vi "Replace Channel.vi"(6 "Index":i32, 7 "Display State In":T1={"Current Channels Info"=[], "Help Prefix"="", "Max Display Size"=8, "Max Size"=0, "Show Buttons"=TRUE, "Data Valid"=refnum, "Show Range"=FALSE, "Range Items"=[], "Range Index"=[]}, 8 "error in (no error)":errorcluster, 9 "New Channels View":T7[](array[typedef]), 10 "Old Channels View":T7[](array[typedef]), 11 "Channels In":T4) -> (0 "error out":errorcluster, 3 "Channels Out":T4, 5 "Display State Out":T1={"Current Channels Info"=[], "Help Prefix"="", "Max Display Size"=8, "Max Size"=0, "Show Buttons"=TRUE, "Data Valid"=refnum, "Show Range"=FALSE, "Range Items"=[], "Range Index"=[]})   [LabVIEW 2021, in "myRIO Channel List.xctl"]
uses:
  <vilib>/myRIO/Common/Express VI Framework/xctls/myRIO Channel List/myRIO Channel List.xctl
  <vilib>/myRIO/Common/Express VI Framework/xctls/myRIO Channel List/typedefs/Channel View.ctl
  <vilib>/myRIO/Common/Express VI Framework/xctls/myRIO Channel List/typedefs/Error Icon.ctl
  <vilib>/myRIO/Common/Express VI Framework/xctls/myRIO Channel List/typedefs/Remove Channel.ctl
  <vilib>/myRIO/Common/Express VI Framework/xctls/myRIO Channel List/State.ctl
  <vilib>/myRIO/Common/Profile Manager Framework/typedefs/Channel Info.ctl
  <vilib>/myRIO/Common/Express VI Framework/typedefs/Data Validate Ref.ctl
  <vilib>/myRIO/Common/Express VI Framework/xctls/myRIO Channel List/Data.ctl
  <vilib>/myRIO/Common/Express VI Framework/xctls/myRIO Channel List/typedefs/Channel Data.ctl
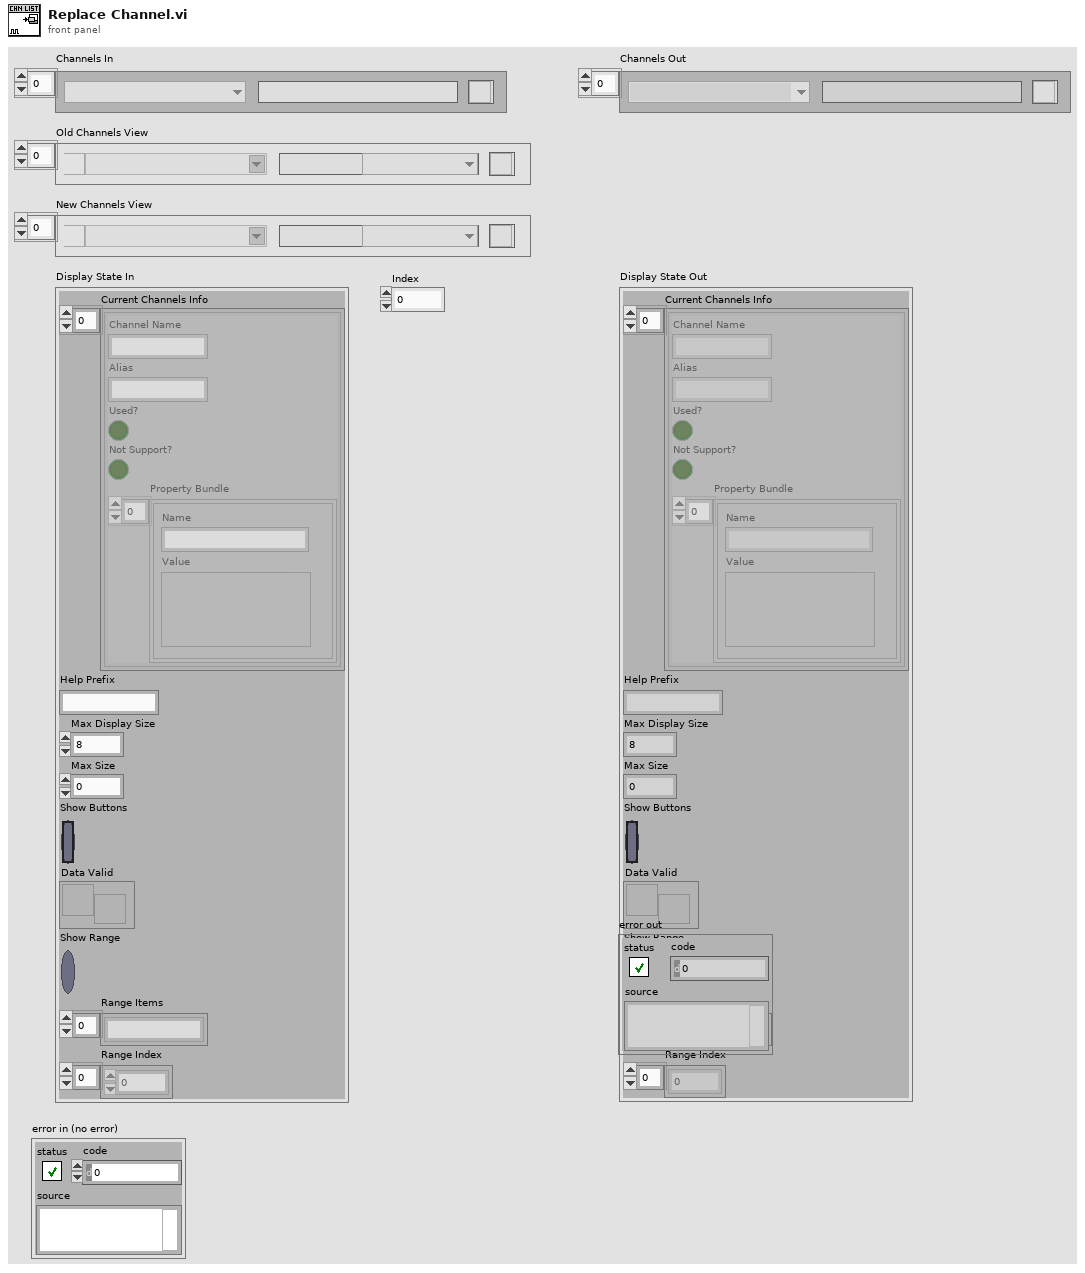
[diagram p1: front panel]
types:
  T1 = typedef "myRIO Channel List.xctl/State.ctl" = cluster{"Current Channels Info":T2[], "Help Prefix":string, "Max Display Size":i32, "Max Size":i32, "Show Buttons":bool, "Data Valid":T3, "Show Range":bool, "Range Items":string[], "Range Index":i32[]}
  T2 = typedef "Channel Info.ctl" = cluster{"Channel Name":string, "Alias":string, "Used?":bool, "Not Support?":bool, "Property Bundle":cluster{"Name":string, "Value":variant}[]}
  T3 = typedef "Data Validate Ref.ctl" = refnum<user-event>
  T4 = typedef "myRIO Channel List.xctl/Data.ctl" = T5[]
  T5 = typedef "myRIO Channel List.xctl/Channel Data.ctl" = cluster{"Channel Name":u16, "Channel Alias":string, "Remove Channel":T6, "Index":i32}
  T6 = typedef "myRIO Channel List.xctl/Remove Channel.ctl" = bool
  T7 = typedef "myRIO Channel List.xctl/Channel View.ctl" = cluster{"Error Icon":T8, "Channel Name":string, "Channel Alias":string, "Remove Channel":T6, "Index":i32, "Range":i32}
  T8 = typedef "myRIO Channel List.xctl/Error Icon.ctl" = bool
  T9 = cluster{"Error Icon":T8, "Channel Name":bool, "Channel Alias":bool, "Remove Channel":T6, "Index":bool, "Range":bool}
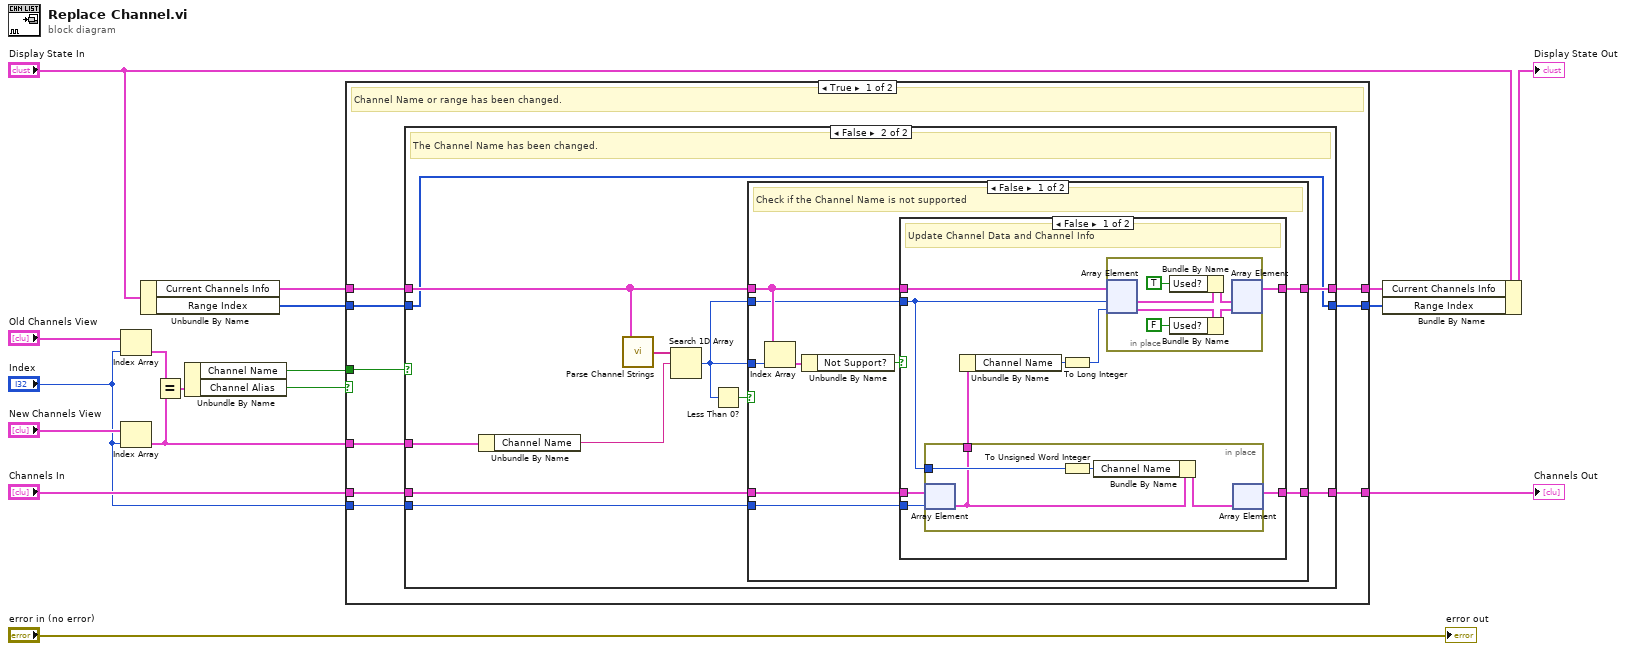
[diagram p0: block diagram]
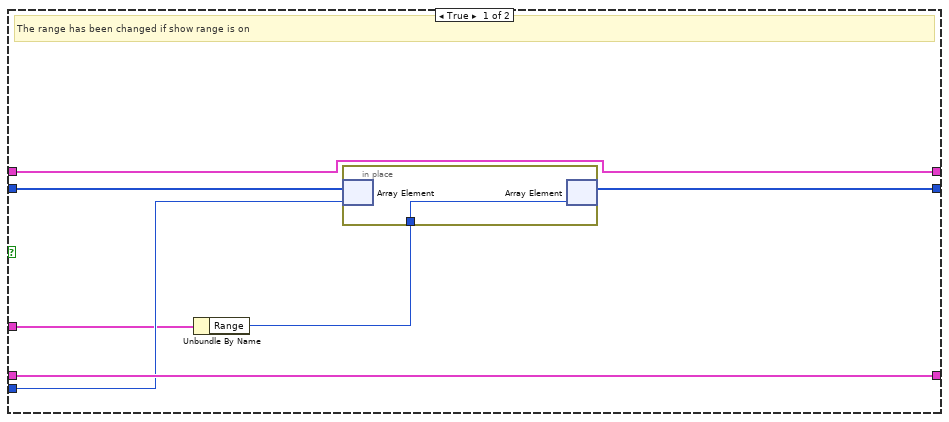
[diagram p2: hidden frame]
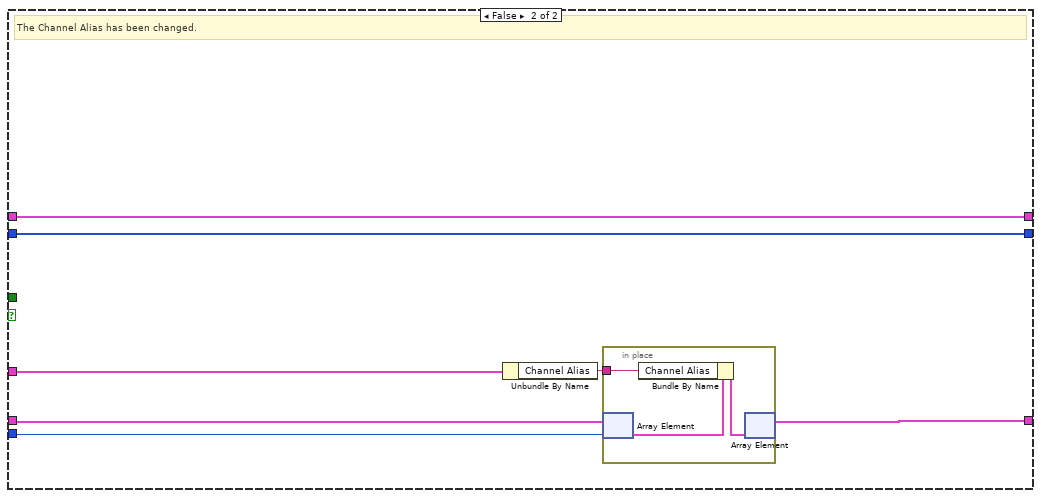
[diagram p5: hidden frame]
diagram:
  n1 = Index Array(array="Old Channels View", index="Index") -> (element=w14:T7)
  n2 = Index Array(array="New Channels View", index="Index") -> (element=w13:T7)
  n3 = Unbundle By Name("Display State In") -> ("Current Channels Info"=w12:T2[], "Range Index"=w4:i32[])
  n4 = Equal?(x=w14, y=w13) -> (x = y?=w15:T9)
  n5 = Unbundle By Name(w15) -> ("Channel Name"=w1:bool, "Channel Alias"=w2:bool)
  n6 = case shown="True" w2 {
    tunnel: w13 -> [w26 w80]
    tunnel: w12 -> [w24 w84]
    tunnel: [w25 w84] -> w11
    tunnel: "Channels In" -> [w23 w83]
    tunnel: "Index" -> [w22 w82]
    tunnel: [w21 w81] -> w6
    tunnel: w1 -> [w20 _]
    tunnel: w4 -> [w19 w78]
    tunnel: [w18 w78] -> w3
    frame True {
      # "Channel Name or range has been changed."
      n7 = case shown="False" w20 {
        tunnel: w26 -> [w30 w45]
        tunnel: [w32 w40] -> w25
        tunnel: w24 -> [w32 w39]
        tunnel: w23 -> [w33 w38]
        tunnel: w22 -> [w31 w37]
        tunnel: [w33 w36] -> w21
        tunnel: w19 -> [w28 w35]
        tunnel: [w27 w35] -> w18
        frame True {
          # "The range has been changed if show range is on"
          n8 = Unbundle By Name(w30) -> ("Range"=w29:i32)
          n9 = in-place {
            in-place-border: w29 -> [w34]
            n10 = in-place-array #1(w28, w31) -> ()  [unwired: 1 out]
            n11 = in-place-array #1(w34) -> (w27:i32[])  [unwired: 1 out]
          }
        }
        frame False {
          # "The Channel Name has been changed."
          n12 = Unbundle By Name(w45) -> ("Channel Name"=w43:string)
          n13 = call <vilib>:"Parse Channel Strings.vi"("Channels Info"=w39) -> ("Channel Strings"=w44:string[])
          n14 = Search 1D Array(1D array=w44, element=w43) -> (index of element=w41:i32)  [unwired: 1 in]
          n15 = Less Than 0?(x=w41) -> (x < 0?=w42:bool)
          n16 = case shown="False" w42 {
            tunnel: w39 -> [w51 w77]
            tunnel: w41 -> [w54 _]
            tunnel: w41 -> [w50 _]
            tunnel: [w49 w77] -> w40
            tunnel: w38 -> [w48 w76]
            tunnel: w37 -> [w47 _]
            tunnel: [w46 w76] -> w36
            frame False {
              # "Check if the Channel Name is not supported"
              n17 = Index Array(array=w51, index=w54) -> (element=w53:T2)
              n18 = Unbundle By Name(w53) -> ("Not Support?"=w52:bool)
              n19 = case shown="False" w52 {
                tunnel: w51 -> [w63 w75]
                tunnel: w50 -> [w59 _]
                tunnel: [w62 w75] -> w49
                tunnel: w48 -> [w61 w74]
                tunnel: w47 -> [w60 _]
                tunnel: [w58 w74] -> w46
                frame False {
                  # "Update Channel Data and Channel Info"
                  n20 = in-place {
                    in-place-border: w59 -> [w66]
                    in-place-border: [w65] -> w56
                    n21 = in-place-array #2(w61, w60) -> (w65:T5)
                    n22 = To Unsigned Word Integer(number=w66) -> (unsigned 16bit integer=w64:u16)
                    n23 = Bundle By Name(cluster=w65, "Channel Name"=w64) -> (w67:T5)
                    n24 = in-place-array #2(w67) -> (w58:T4)  [unwired: 1 out]
                  }
                  n25 = Unbundle By Name(w56) -> ("Channel Name"=w57:u16)
                  n26 = To Long Integer(number=w57) -> (32bit integer=w55:i32)
                  n27 = in-place {
                    n28 = in-place-array #3(w63, w59, w55) -> (w73:T2, w72:T2)
                    n29 = Bundle By Name(cluster=w73, "Used?"=TRUE) -> (w71:T2)
                    n30 = Bundle By Name(cluster=w72, "Used?"=FALSE) -> (w70:T2)
                    n31 = in-place-array #3(w71, w70) -> (w62:T2[])  [unwired: 2 out]
                  }
                }
                frame True {
                  # "Non-supported Channel Name"
                }
              }
            }
            frame True {
              # "Non-supported Channel Name"
            }
          }
        }
      }
    }
    frame False {
      # "The Channel Alias has been changed."
      n32 = Unbundle By Name(w80) -> ("Channel Alias"=w79:string)
      n33 = in-place {
        in-place-border: w79 -> [w85]
        n34 = in-place-array #4(w83, w82) -> (w87:T5)
        n35 = Bundle By Name(cluster=w87, "Channel Alias"=w85) -> (w86:T5)
        n36 = in-place-array #4(w86) -> (w81:T4)  [unwired: 1 out]
      }
    }
  }
  "Channels Out" <- w6
  n37 = Bundle By Name(cluster="Display State In", "Current Channels Info"=w11, "Range Index"=w3) -> (→"Display State Out":T1)
  "error out" <- "error in (no error)"
